vi "Lineup.vi"() -> ()   [LabVIEW 2014]
uses:
  Begin/Global RefNums.vi
  <vilib>/Rock Robotics/WPI/Ultrasonic/WPI_SonarMB1010AnalogRefNum Registry Get.vi
  Begin/Global Variables.vi
  <vilib>/Rock Robotics/WPI/Ultrasonic/WPI_SonarMB1010AnalogGetRange.vi
  <vilib>/addons/control/pid/NI_PID_pid.lvlib
  <vilib>/addons/control/pid/pid.llb/PID (DBL).vi
panel:
  in  "Turn Speed":dbl=0.35
  in  "Distance Buffer":dbl=1.1
  in  "Strafe Speed":dbl=-0.35
  in  "Distance":dbl=12.0
  in  "Angle Buffer":dbl=1.5
  in  "milliseconds to wait":u32=100
  in  "lower limit":dbl=0.2
  in  "Average Num":dbl=10.0 format="%#_13g"
  in  "Deadband":dbl
  in  "Angle PID gains":T1={"proportional gain (Kc)"=0.11, "integral time (Ti, min)"=0.1, "derivative time (Td, min)"=0.0} {"derivative time (Td, min)" format="%.3f"; "integral time (Ti, min)" format="%.3f"; "proportional gain (Kc)" format="%.3f"}
  in  "Angle output range":cluster{"output high":dbl, "output low":dbl}={"output high"=0.75, "output low"=-0.75} {"output low" format="%.2f"; "output high" format="%.2f"}
  in  "Forward Output Range":cluster{"output high":dbl, "output low":dbl}={"output high"=1.0, "output low"=-1.0} {"output low" format="%.2f"; "output high" format="%.2f"}
  in  "Forward PID gains":T1={"proportional gain (Kc)"=0.1, "integral time (Ti, min)"=0.147, "derivative time (Td, min)"=0.0} {"derivative time (Td, min)" format="%.3f"; "integral time (Ti, min)" format="%.3f"; "proportional gain (Kc)" format="%.3f"}
  in  "Forward Range":dbl=0.3
  in  "Forward":dbl=12.0 format="%.2f"
  in  "Angle Range":dbl=0.5 format="%#_13g"
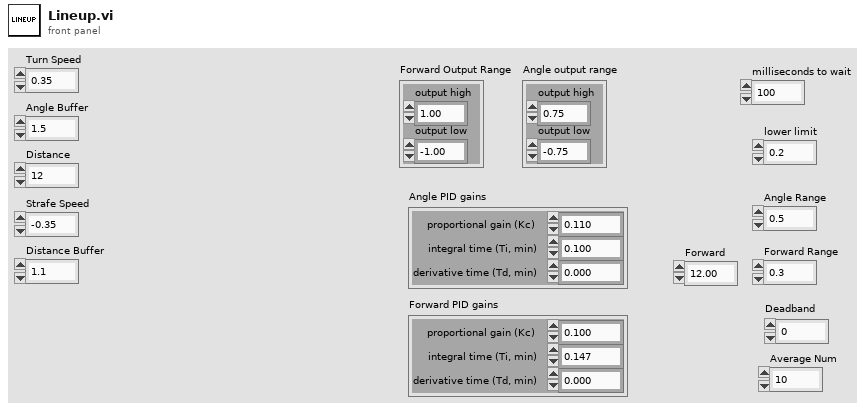
[diagram p1: front panel]
types:
  T1 = cluster{"proportional gain (Kc)":dbl, "integral time (Ti, min)":dbl, "derivative time (Td, min)":dbl}
  T2 = typedef "WPI_SonarMB1010AnalogDeviceRef.ctl" = cluster{"AIDeviceRef":T3, "Scaling factor (V/in)":dbl, "Average Bits":u8}
  T3 = typedef "WPI_AnalogChannelDevRef.ctl" = cluster{"DevStatus":errorcluster, "Controller":T4, "Analog Channel":T5}
  T4 = typedef "FPGA_TypedefAnalogModule.ctl" = enum16{"Controller 1"}
  T5 = typedef "FPGA_AIChannel.ctl" = enum8{"AI 0", "AI 1", "AI 2", "AI 3", "AI MXP 0", "AI MXP 1", "AI MXP 2", "AI MXP 3", "Invalid"}
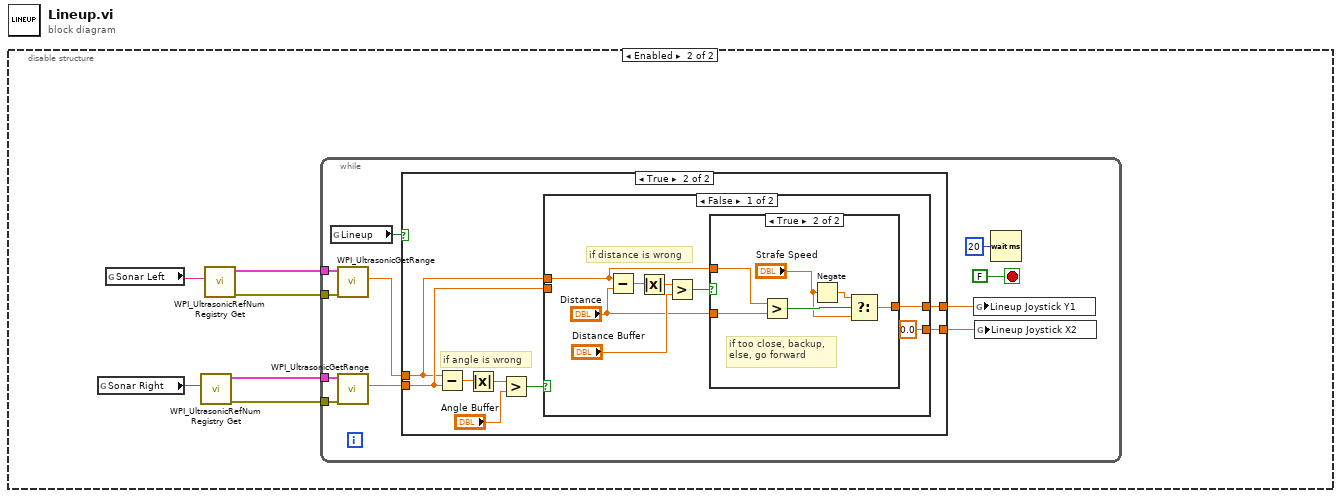
[diagram p0: block diagram]
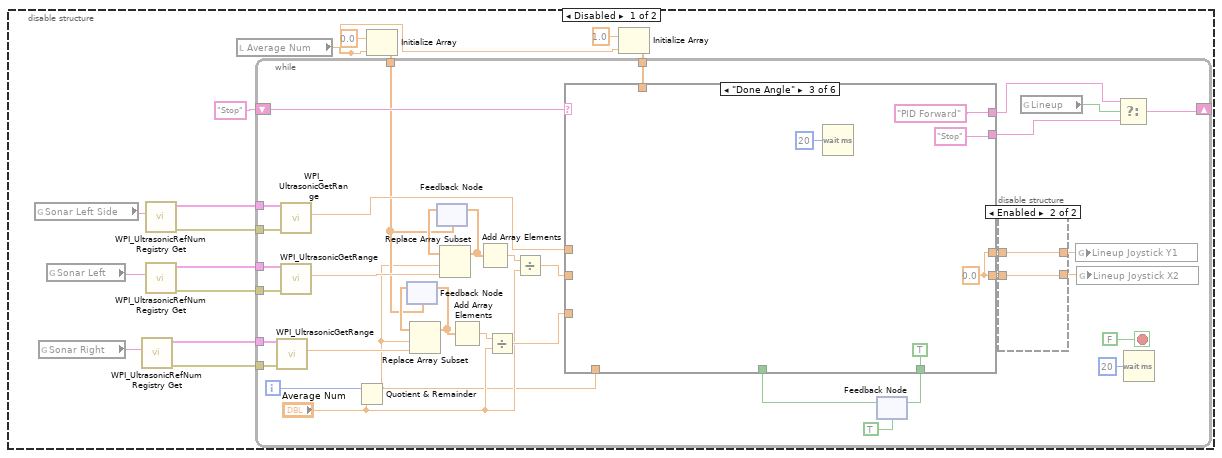
[diagram p2: hidden frame]
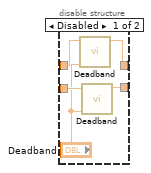
[diagram p3: hidden frame]
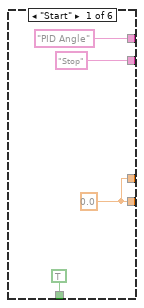
[diagram p4: hidden frame]
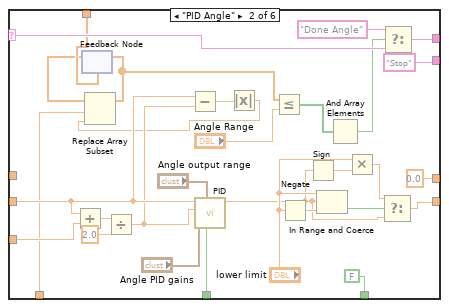
[diagram p5: hidden frame]
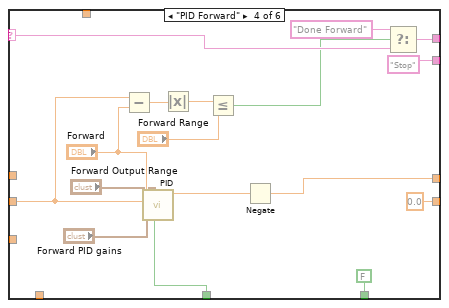
[diagram p6: hidden frame]
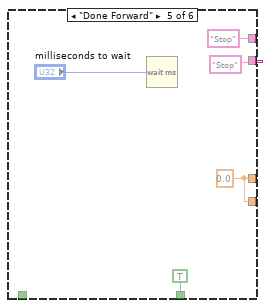
[diagram p7: hidden frame]
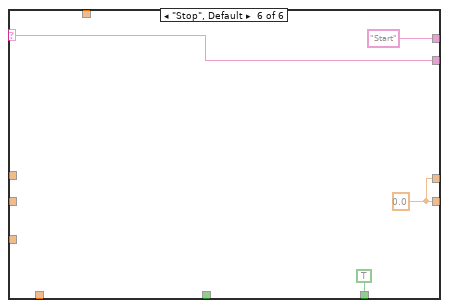
[diagram p8: hidden frame]
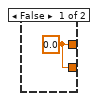
[diagram p9: hidden frame]
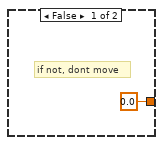
[diagram p10: hidden frame]
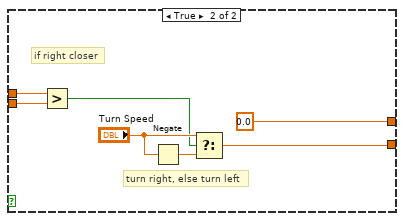
[diagram p11: hidden frame]
diagram:
  n1 = disable-structure shown="Enabled" {
    frame Disabled {
      n2 = global read "Global RefNums.vi" "Sonar Left Side"() -> (w8:string)
      n3 = global read "Global RefNums.vi" "Sonar Right"() -> (w10:string)
      n4 = global read "Global RefNums.vi" "Sonar Left"() -> (w9:string)
      n5 = call-poly <vilib>:"WPI_UltrasonicRefNum Registry Get.vi"("refnum name"=w10) -> ("error out"=w12:errorcluster, "SonarMB1010AnalogDevRef"=w11:T2)  [unwired: 9 in]
      n6 = call-poly <vilib>:"WPI_UltrasonicRefNum Registry Get.vi"("refnum name"=w8) -> ("error out"=w7:errorcluster, "SonarMB1010AnalogDevRef"=w6:T2)  [unwired: 9 in]
      n7 = call-poly <vilib>:"WPI_UltrasonicRefNum Registry Get.vi"("refnum name"=w9) -> ("error out"=w13:errorcluster, "SonarMB1010AnalogDevRef"=w14:T2)  [unwired: 9 in]
      n8 = local read "Average Num"() -> (w1:dbl)
      n9 = Initialize Array(0.0 ("element"), w1) -> (w5:dbl[])
      n10 = Initialize Array(1.0 ("element"), w1) -> (w2:dbl[])
      n11 = while {
        shift-right: [w44] -> _
        shift-left: "Stop" -> [w50]
        tunnel: w14 -> [w49]
        tunnel: w13 -> [w48]
        tunnel: w11 -> [w46]
        tunnel: w12 -> [w47]
        tunnel: w6 -> [w39]
        tunnel: w7 -> [w40]
        tunnel: w5 -> [w22]
        tunnel: w2 -> [w18]
        i -> [w33]
        stop <- FALSE stop-if-true
        n12 = call-poly <vilib>:"WPI_UltrasonicGetRange.vi"("error in"=w47, "SonarMB1010AnalogDevRef"=w46) -> ("Distance"=w24:dbl)  [unwired: 7 in, 2 out]
        n13 = call-poly <vilib>:"WPI_UltrasonicGetRange.vi"("error in"=w40, "SonarMB1010AnalogDevRef"=w39) -> ("Distance"=w38:dbl)  [unwired: 7 in, 2 out]
        n14 = call-poly <vilib>:"WPI_UltrasonicGetRange.vi"("error in"=w48, "SonarMB1010AnalogDevRef"=w49) -> ("Distance"=w23:dbl)  [unwired: 7 in, 2 out]
        n15 = Quotient & Remainder(x=w33, y="Average Num") -> (x-y*floor(x/y)=w16:dbl)  [unwired: 1 out]
        n16 = feedback #1(w22) -> (w26:dbl[])
        n17 = Replace Array Subset(array=w26, new element=w24, index=w16) -> (w27:dbl[])
        n18 = feedback-in #1(w27) -> ()
        n19 = feedback #2(w22) -> (w30:dbl[])
        n20 = Replace Array Subset(array=w30, new element=w23, index=w16) -> (w31:dbl[])
        n21 = feedback-in #2(w31) -> ()
        n22 = Add Array Elements(numeric array=w27) -> (sum=w28:dbl)
        n23 = Add Array Elements(numeric array=w31) -> (sum=w32:dbl)
        n24 = Divide(x=w28, y="Average Num") -> (x/y=w25:dbl)
        n25 = Divide(x=w32, y="Average Num") -> (x/y=w29:dbl)
        n26 = feedback #3(TRUE) -> (w21:bool)
        n27 = case shown="\"Done Angle\"" w50 {
          selector: w50 -> [_ w90 _ w109 _ w122]
          tunnel: ["PID Angle" ("t") w89 "PID Forward" ("t") w108 "Stop" ("t") "Start" ("t")] -> w43
          tunnel: [w62 0.0 ("Lineup Joystick X2") w94 w100 w118 w123] -> w37
          tunnel: [w62 w63 w94 0.0 ("Lineup Joystick X2") w118 w123] -> w35
          tunnel: w29 -> [_ w83 _ w112 _ _]
          tunnel: w25 -> [_ w82 _ _ _ _]
          tunnel: ["Stop" ("t") "Stop" ("t") "Stop" ("t") "Stop" ("t") "Stop" ("t") w122] -> w42
          tunnel: w38 -> [_ _ _ _ _ _]
          tunnel: w21 -> [_ w78 _ w98 _ _]
          tunnel: [TRUE FALSE TRUE FALSE TRUE TRUE] -> w19
          tunnel: w18 -> [_ w76 _ _ _ _]
          tunnel: w16 -> [_ w74 _ _ _ _]
          frame "Start" {
            w62 = 0.0 ("Lineup Joystick X2")
          }
          frame "PID Angle" {
            n28 = Add(x=w83, y=w82) -> (x+y=w81:dbl)
            n29 = feedback #4(w76) -> (w75:dbl[])
            n30 = Divide(x=w81, y=2.0) -> (x/y=w79:dbl)
            n31 = Subtract(x=w83, y=w79) -> (x-y=w92:dbl)
            n32 = call-poly <vilib>:"PID.vi"("reinitialize? (F)"=w78, "output range"="Angle output range", "PID gains"="Angle PID gains", "process variable"=w79, "setpoint"=w83) -> ("output"=w64:dbl)  [unwired: 5 in, 1 out]
            n33 = Absolute Value(x=w92) -> (abs(x)=w73:dbl)
            n34 = Replace Array Subset(array=w75, new element=w73, index=w74) -> (w72:dbl[])
            n35 = feedback-in #4(w72) -> ()
            n36 = Less Or Equal?(x=w72, y="Angle Range") -> (x <= y?=w71:bool[])
            n37 = Negate(x="lower limit") -> (-x=w69:dbl)
            n38 = Sign(1:w64) -> (0:w67:dbl)
            n39 = In Range and Coerce(upper limit="lower limit", x=w64, lower limit=w69) -> (In Range?=w68:bool)  [unwired: 1 out]
            n40 = And Array Elements(Boolean array=w71) -> (logical AND=w70:bool)
            n41 = Multiply(x="lower limit", y=w67) -> (x*y=w65:dbl)
            n42 = Select(t=w65, s=w68, f=w64) -> (s? t:f=w63:dbl)
            n43 = Select(t="Done Angle", s=w70, f=w90) -> (s? t:f=w89:string)
          }
          frame "Done Angle" {
            w94 = 0.0 ("Lineup Joystick X2")
            n44 = Wait (ms)(milliseconds to wait=u32 20) -> ()  [unwired: 1 out]
          }
          frame "PID Forward" {
            n45 = Subtract(x=w112, y="Forward") -> (x-y=w114:dbl)
            n46 = call-poly <vilib>:"PID.vi"("reinitialize? (F)"=w98, "output range"="Forward Output Range", "PID gains"="Forward PID gains", "process variable"=w112, "setpoint"="Forward") -> ("output"=w101:dbl)  [unwired: 5 in, 1 out]
            n47 = Absolute Value(x=w114) -> (abs(x)=w113:dbl)
            n48 = Less Or Equal?(x=w113, y="Forward Range") -> (x <= y?=w107:bool)
            n49 = Negate(x=w101) -> (-x=w100:dbl)
            n50 = Select(t="Done Forward", s=w107, f=w109) -> (s? t:f=w108:string)
          }
          frame "Done Forward" {
            w118 = 0.0 ("Lineup Joystick X2")
            n51 = Wait (ms)(milliseconds to wait="milliseconds to wait") -> ()  [unwired: 1 out]
          }
          frame "Stop", Default {
            w123 = 0.0 ("Lineup Joystick X2")
          }
        }
        n52 = feedback-in #3(w19) -> ()
        n53 = disable-structure shown="Enabled" {
          disable-tunnel: w37 -> [w56 w58]
          disable-tunnel: [w55 w58] -> w36
          disable-tunnel: w35 -> [w54 w57]
          disable-tunnel: [w53 w57] -> w34
          frame Disabled {
            n54 = call "Deadband.vi"("Value to Deadband (default of 0.1)"="Deadband", "Value"=w56) -> ("Deadbanded Value"=w55:dbl)  [unwired: 9 in]
            n55 = call "Deadband.vi"("Value to Deadband (default of 0.1)"="Deadband", "Value"=w54) -> ("Deadbanded Value"=w53:dbl)  [unwired: 9 in]
          }
          frame Enabled {
          }
        }
        n56 = global read "Global Variables.vi" "Lineup"() -> (w41:bool)
        n57 = global write "Global Variables.vi" "Lineup Joystick Y1"(w36) -> ()
        n58 = global write "Global Variables.vi" "Lineup Joystick X2"(w34) -> ()
        n59 = Select(t=w43, s=w41, f=w42) -> (s? t:f=w44:string)
        n60 = Wait (ms)(milliseconds to wait=u32 20) -> ()  [unwired: 1 out]
      }
    }
    frame Enabled {
      n61 = global read "Global RefNums.vi" "Sonar Right"() -> (w129:string)
      n62 = global read "Global RefNums.vi" "Sonar Left"() -> (w128:string)
      n63 = call-poly <vilib>:"WPI_UltrasonicRefNum Registry Get.vi"("refnum name"=w129) -> ("error out"=w124:errorcluster, "SonarMB1010AnalogDevRef"=w125:T2)  [unwired: 9 in]
      n64 = call-poly <vilib>:"WPI_UltrasonicRefNum Registry Get.vi"("refnum name"=w128) -> ("error out"=w126:errorcluster, "SonarMB1010AnalogDevRef"=w127:T2)  [unwired: 9 in]
      n65 = while {
        tunnel: w127 -> [w138]
        tunnel: w126 -> [w137]
        tunnel: w125 -> [w140]
        tunnel: w124 -> [w139]
        stop <- FALSE stop-if-true
        n66 = global read "Global Variables.vi" "Lineup"() -> (w130:bool)
        n67 = call-poly <vilib>:"WPI_UltrasonicGetRange.vi"("error in"=w137, "SonarMB1010AnalogDevRef"=w138) -> ("Distance"=w133:dbl)  [unwired: 7 in, 2 out]
        n68 = call-poly <vilib>:"WPI_UltrasonicGetRange.vi"("error in"=w139, "SonarMB1010AnalogDevRef"=w140) -> ("Distance"=w134:dbl)  [unwired: 7 in, 2 out]
        n69 = case shown="True" w130 {
          tunnel: w134 -> [_ w145]
          tunnel: w133 -> [_ w144]
          tunnel: [w141 w143] -> w132
          tunnel: [w141 w142] -> w131
          frame False {
            w141 = 0.0 ("Strafe Speed")
          }
          frame True {
            # "if angle is wrong"
            n70 = Subtract(x=w144, y=w145) -> (x-y=w149:dbl)
            n71 = Absolute Value(x=w149) -> (abs(x)=w148:dbl)
            n72 = Greater?(x=w148, y="Angle Buffer") -> (0:w146:bool)
            n73 = case shown="False" w146 {
              tunnel: w145 -> [_ w171]
              tunnel: w144 -> [w155 w170]
              tunnel: [w156 0.0 ("Strafe Speed")] -> w143
              tunnel: [0.0 ("Turn Speed") w168] -> w142
              frame False {
                # "if distance is wrong"
                n74 = Subtract(x=w155, y="Distance") -> (x-y=w154:dbl)
                n75 = Absolute Value(x=w154) -> (abs(x)=w153:dbl)
                n76 = Greater?(x=w153, y="Distance Buffer") -> (0:w152:bool)
                n77 = case shown="True" w152 {
                  tunnel: [0.0 ("Strafe Speed") w164] -> w156
                  tunnel: w155 -> [_ w162]
                  tunnel: "Distance" -> [_ w161]
                  frame False {
                    # "if not, dont move"
                  }
                  frame True {
                    # "if too close, backup,\nelse, go forward"
                    n78 = Greater?(x=w162, y=w161) -> (0:w163:bool)
                    n79 = Negate(x="Strafe Speed") -> (-x=w160:dbl)
                    n80 = Select(t=w160, s=w163, f="Strafe Speed") -> (s? t:f=w164:dbl)
                  }
                }
              }
              frame True {
                # "turn right, else turn left"
                # "if right closer"
                n81 = Greater?(x=w170, y=w171) -> (0:w165:bool)
                n82 = Negate(x="Turn Speed") -> (-x=w167:dbl)
                n83 = Select(t="Turn Speed", s=w165, f=w167) -> (s? t:f=w168:dbl)
              }
            }
          }
        }
        n84 = global write "Global Variables.vi" "Lineup Joystick Y1"(w132) -> ()
        n85 = global write "Global Variables.vi" "Lineup Joystick X2"(w131) -> ()
        n86 = Wait (ms)(milliseconds to wait=u32 20) -> ()  [unwired: 1 out]
      }
    }
  }
